vi "Update_Inlet_Temp_Profile.vi"(3 "Mode":T5, 5 "Traverse line In":T2 {"Carrier_2 Q (l/min)" format="%#.2f"; "Row Duration (mins)" format="%#.1f"; "Row No" min=0; "Trace Gas Concentration (%)" min=0.0 format="%#_4f"; "Carrier_1 Q (l/min)" format="%#.2f"; "Tunnel Speed" format="%#.2f"; "Start X" format="%#.2f"; "Start Y" format="%#.2f"; "Start Z" format="%#.2f"; "End X" format="%#.2f"; "End Y" format="%#.2f"; "End Z" format="%#.2f"; "Averaging time (min)" min=0.0 format="%#.2f"}) -> (0 "Error Message":string, 1 "Status":T1, 2 "Traverse line Out":T2 {"Carrier_2 Q (l/min)" format="%#.2f"; "Row Duration (mins)" format="%#.1f"; "Row No" min=0; "Trace Gas Concentration (%)" min=0.0 format="%#_4f"; "Carrier_1 Q (l/min)" format="%#.2f"; "Tunnel Speed" format="%#.2f"; "Start X" format="%#.2f"; "Start Y" format="%#.2f"; "Start Z" format="%#.2f"; "End X" format="%#.2f"; "End Y" format="%#.2f"; "End Z" format="%#.2f"; "Averaging time (min)" min=0.0 format="%#.2f"})   [LabVIEW 2015]
uses:
  Gen Trav/Traverse_cluster.ctl
  Gen Trav/Spacing.ctl
  Controls/Multi_run_mode.ctl
  Controls/User_Specific_mode.ctl
  Gen Trav/Multi_Run_Status.ctl
  <vilib>/Analysis/baseanly.llb/Mean (DBL).vi
  <vilib>/Analysis/NI_AALBase.lvlib
panel:
  out "Set Values":dbl[](array[numeric])
  out "Sub set":string[](array[string])=["EnFlo_Tunnel:Temp:Inlet_Y=0_Z=50", "EnFlo_Tunnel:Temp:Inlet_Y=0_Z=150", "EnFlo_Tunnel:Temp:Inlet_Y=0_Z=250", "EnFlo_Tunnel:Temp:Inlet_Y=0_Z=350", "EnFlo_Tunnel:Temp:Inlet_Y=0_Z=450", "EnFlo_Tunnel:Temp:Inlet_Y=0_Z=550", "EnFlo_Tunnel:Temp:Inlet_Y=0_Z=650", "EnFlo_Tunnel:Temp:Inlet_Y=0_Z=750", "EnFlo_Tunnel:Temp:Inlet_Y=0_Z=850", "EnFlo_Tunnel:Temp:Inlet_Y=0_Z=950", "EnFlo_Tunnel:Temp:Inlet_Y=0_Z=1050", "EnFlo_Tunnel:Temp:Inlet_Y=0_Z=1150", "EnFlo_Tunnel:Temp:Inlet_Y=0_Z=1250", "EnFlo_Tunnel:Temp:Inlet_Y=0_Z=1350", "EnFlo_Tunnel:Temp:Inlet_Y=0_Z=1450", "EnFlo_Tunnel:Chilled Water:Dem Temp"]
  out "Chilled water Dem Temp":dbl
  # "X           Y            Z"
  # "Start"
  # "End"
  # "X           Y            Z"
  # "Start"
  # "End"
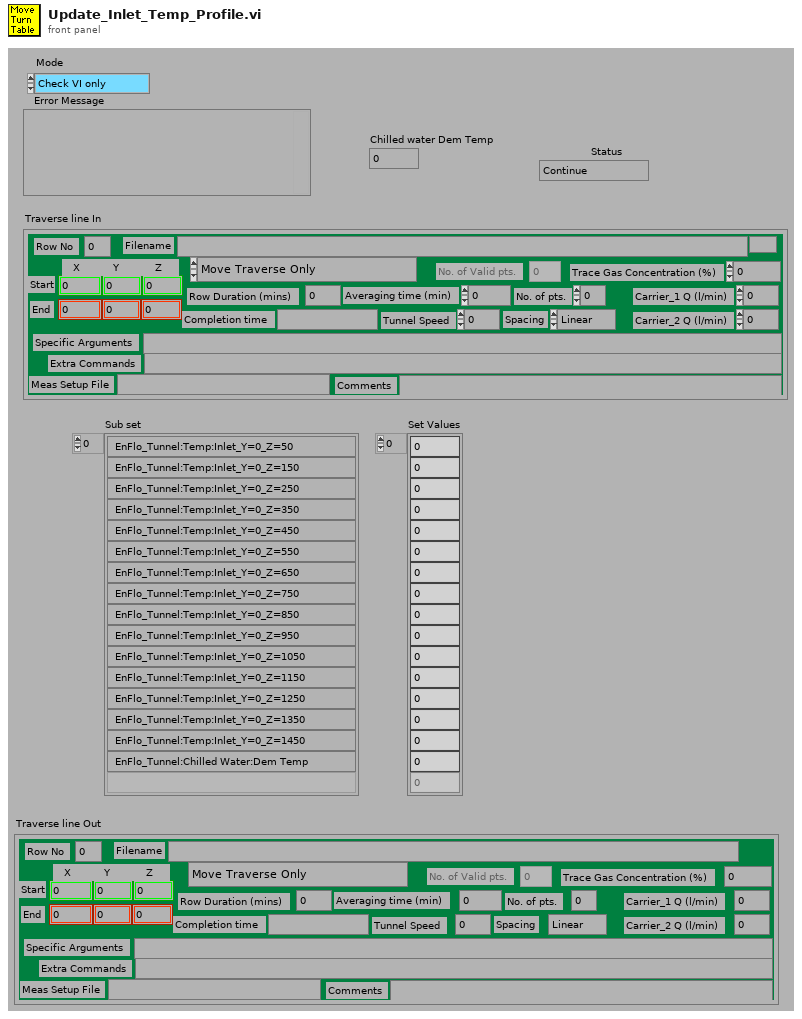
[diagram p1: front panel]
types:
  T1 = typedef "Multi_Run_Status.ctl" = enum16{"Continue", "Jump to Next Point", "Jump to Next Row", "Jump To Fall Back", "Terminate Run"}
  T2 = typedef "Traverse_cluster.ctl" = cluster{"Start X":sgl, "Start Y":sgl, "Start Z":sgl, "End X":sgl, "End Y":sgl, "End Z":sgl, "No. of pts.":i32, "Spacing":T3, "Filename":path, "Tunnel Speed":dbl, "Averaging time (min)":dbl, "Extra Commands":string, "Carrier_1 Q (l/min)":dbl, "Carrier_2 Q (l/min)":dbl, "Trace Gas Concentration (%)":dbl, "Specific Arguments":string, "Comments":string, "Row No":i32, "Row Type Selector":T4, "Completion time":string, "Row Duration (mins)":dbl, "No. of Valid pts.":i32, "Meas Setup File":string}
  T3 = typedef "Spacing.ctl" = enum16{"Linear", "Log", "Gauss", "Specified", "N/A"}
  T4 = typedef "Multi_run_mode.ctl" = enum16{"Move Traverse Only", "Set Tunnel Speed Only", "Set Source Only", "Set Measurement Conditions", "Single Measurement", "Vertical Profile", "Lateral Profile", "Longitudinal Profile", "Explore Volume", "Multi-Axis Profile", "Auto Calibrate", "Meas Fast FID Bkgnd", "Check Beam Power", "Scanning Valve Measurement", "Run VI Named:", "Set ADAM Ch", "Wait (minutes)", "Send Message", "Synchronize With:", "Fall Back to this Row", "Turn Off Row Repeating", "Blank Row", "Traverse 3D Volume"}
  T5 = typedef "User_Specific_mode.ctl" = enum16{"Check VI only", "Run VI"}
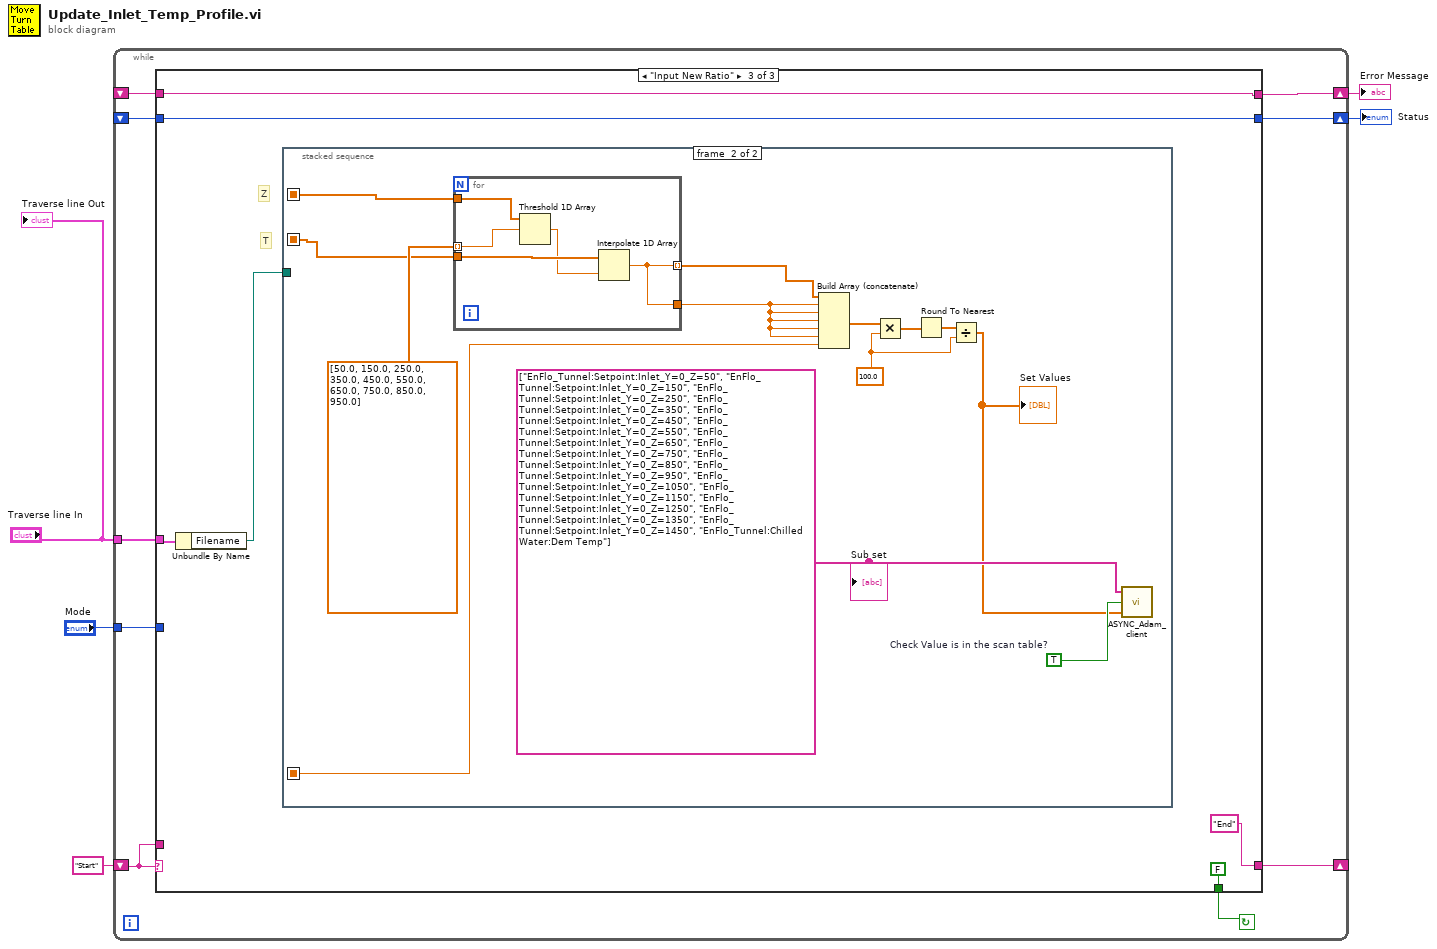
[diagram p0: block diagram]
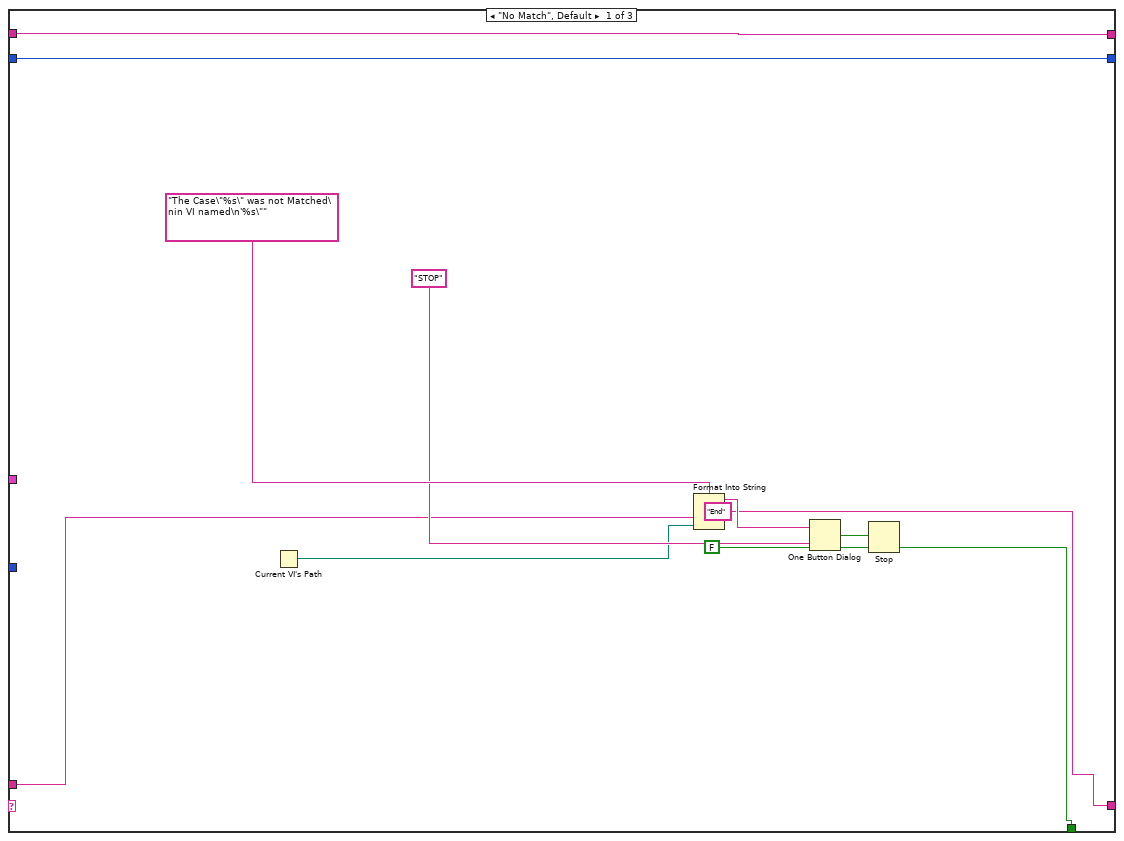
[diagram p2: hidden frame]
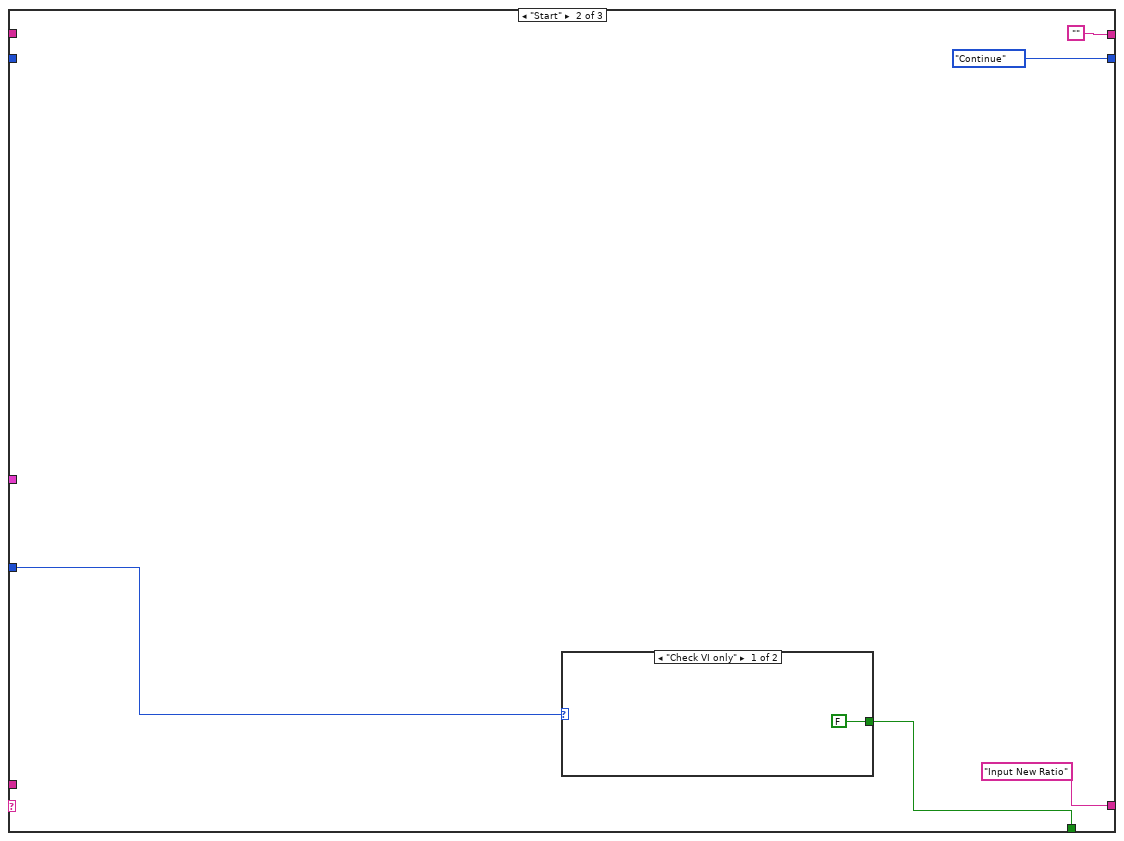
[diagram p3: hidden frame]
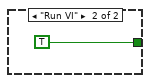
[diagram p4: hidden frame]
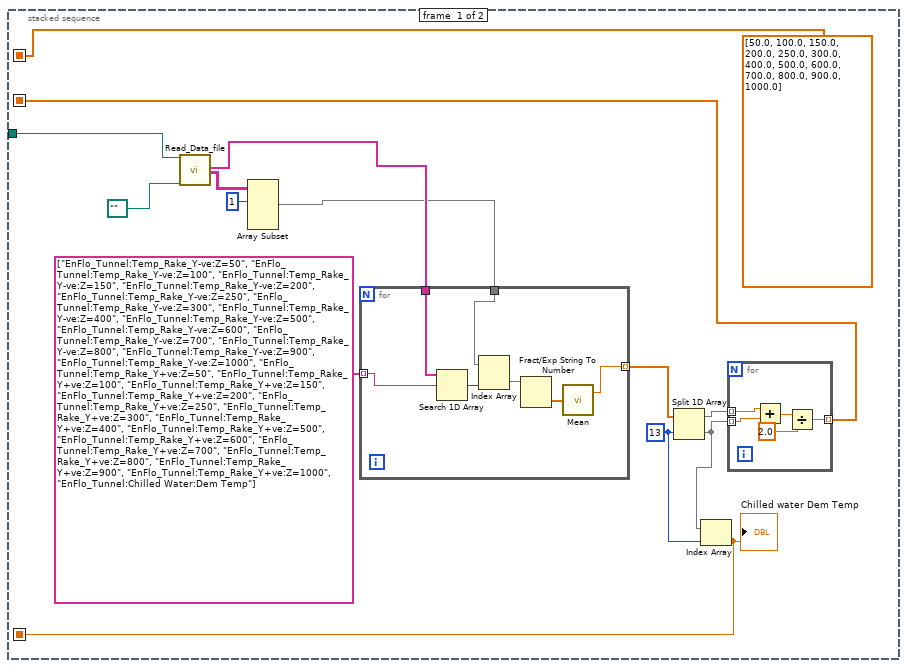
[diagram p5: hidden frame]
diagram:
  n1 = while {
    shift-left: _ -> [w7]
    shift-right: [w6] -> w2
    shift-left: _ -> [w10]
    shift-right: [w8] -> w3
    tunnel: "Traverse line In" -> [w13]
    tunnel: "Mode" -> [w14]
    shift-left: "Start" -> [w9]
    shift-right: [w11] -> _
    stop <- w12 continue-if-true
    n2 = case shown="\"Input New Ratio\"" w9 {
      tunnel: w13 -> [_ _ w35]
      tunnel: w14 -> [_ w28 _]
      tunnel: [FALSE ("Update Datum Powers?") w27 FALSE ("Update Datum Powers?")] -> w12
      tunnel: ["End" "Input New Ratio" "End"] -> w11
      tunnel: w10 -> [w19 _ w36]
      tunnel: [w19 "" w36] -> w8
      tunnel: w9 -> [w16 _ _]
      tunnel: w7 -> [w15 _ w37]
      tunnel: [w15 Multi_Run_Status."Continue" ("Status") w37] -> w6
      frame "No Match", Default {
        n3 = Current VI's Path() -> (path=w20:path)
        n4 = Format Into String(format string="The Case\"%s\" was not Matched\nin VI named\n'%s\"" ("Format String"), w16, w20) -> (resulting string=w23:string)  [unwired: 2 in, 1 out]
        n5 = One Button Dialog(message=w23, button name ("OK")="STOP") -> (true=w21:bool)
        n6 = Stop(stop? (T)=w21) -> ()
      }
      frame "Start" {
        n7 = case shown="\"Check VI only\"" w28 {
          tunnel: [FALSE ("Update Datum Powers?") TRUE ("Update Datum Powers?")] -> w27
          frame "Check VI only" {
          }
          frame "Run VI" {
          }
        }
      }
      frame "Input New Ratio" {
        # "T"
        # "Z"
        n8 = Unbundle By Name(w35) -> ("Filename"=w34:path)
        n9 = stacked-sequence {
          seq-local: [dbl[] [50.0, 100.0, 150.0, 200.0, 250.0, 300.0, 400.0, 500.0, 600.0, 700.0, 800.0, 900.0, 1000.0] ("second subarray") _] -> [_ w76]
          seq-local: [w42 _] -> [_ w74]
          seq-local: [w38 _] -> [_ w69]
          tunnel: w34 -> [w41 _]
          frame #0 {
            w39 = 13 ("index")
            n10 = call "Read_Data_file.vi"("Results file"=w41, "Template File"=path "") -> ("Ch names Out"=w50:string[], "Channel Values Out"=w48:string[][])  [unwired: 3 in, 13 out]
            n11 = Array Subset(array=w48, index (row)=1 ("index")) -> (w46:string[][])  [unwired: 3 in]
            n12 = for {
              tunnel: w50 -> [w63]
              tunnel: string[] ["EnFlo_Tunnel:Temp_Rake_Y-ve:Z=50", "EnFlo_Tunnel:Temp_Rake_Y-ve:Z=100", "EnFlo_Tunnel:Temp_Rake_Y-ve:Z=150", "EnFlo_Tunnel:Temp_Rake_Y-ve:Z=200", "EnFlo_Tunnel:Temp_Rake_Y-ve:Z=250", "EnFlo_Tunnel:Temp_Rake_Y-ve:Z=300", "EnFlo_Tunnel:Temp_Rake_Y-ve:Z=400", "EnFlo_Tunnel:Temp_Rake_Y-ve:Z=500", "EnFlo_Tunnel:Temp_Rake_Y-ve:Z=600", "EnFlo_Tunnel:Temp_Rake_Y-ve:Z=700", "EnFlo_Tunnel:Temp_Rake_Y-ve:Z=800", "EnFlo_Tunnel:Temp_Rake_Y-ve:Z=900", "EnFlo_Tunnel:Temp_Rake_Y-ve:Z=1000", "EnFlo_Tunnel:Temp_Rake_Y+ve:Z=50", "EnFlo_Tunnel:Temp_Rake_Y+ve:Z=100", "EnFlo_Tunnel:Temp_Rake_Y+ve:Z=150", "EnFlo_Tunnel:Temp_Rake_Y+ve:Z=200", "EnFlo_Tunnel:Temp_Rake_Y+ve:Z=250", "EnFlo_Tunnel:Temp_Rake_Y+ve:Z=300", "EnFlo_Tunnel:Temp_Rake_Y+ve:Z=400", "EnFlo_Tunnel:Temp_Rake_Y+ve:Z=500", "EnFlo_Tunnel:Temp_Rake_Y+ve:Z=600", "EnFlo_Tunnel:Temp_Rake_Y+ve:Z=700", "EnFlo_Tunnel:Temp_Rake_Y+ve:Z=800", "EnFlo_Tunnel:Temp_Rake_Y+ve:Z=900", "EnFlo_Tunnel:Temp_Rake_Y+ve:Z=1000", "EnFlo_Tunnel:Chilled Water:Dem Temp"] ("Sub set") -> [w62] mode=indexing
              tunnel: w46 -> [w61]
              tunnel: [w57] -> w45 mode=indexing
              n13 = Search 1D Array(1D array=w63, element=w62) -> (index of element=w60:i32)  [unwired: 1 in]
              n14 = Index Array(array=w61, index (col)=w60) -> (element=w59:string[])  [unwired: 1 in]
              n15 = Fract/Exp String To Number(string=w59) -> (number=w58:dbl[])  [unwired: 3 in, 1 out]
              n16 = call-poly <vilib>:"Mean.vi"("X"=w58) -> ("mean"=w57:dbl)  [unwired: 1 out]
            }
            n17 = Split 1D Array(array=w45, index=w39) -> (first subarray=w44:dbl[], second subarray=w40:dbl[])
            n18 = Index Array(array=w40, index=w39) -> (element=w38:dbl)
            "Chilled water Dem Temp" <- w38
            n19 = for {
              tunnel: w44 -> [w56] mode=indexing
              tunnel: w40 -> [w55] mode=indexing
              tunnel: [w52] -> w42 mode=indexing
              n20 = Add(x=w56, y=w55) -> (x+y=w54:dbl)
              n21 = Divide(x=w54, y=2.0) -> (x/y=w52:dbl)
            }
          }
          frame #1 {
            w65 = 100.0
            w70 = string[] ["EnFlo_Tunnel:Setpoint:Inlet_Y=0_Z=50", "EnFlo_Tunnel:Setpoint:Inlet_Y=0_Z=150", "EnFlo_Tunnel:Setpoint:Inlet_Y=0_Z=250", "EnFlo_Tunnel:Setpoint:Inlet_Y=0_Z=350", "EnFlo_Tunnel:Setpoint:Inlet_Y=0_Z=450", "EnFlo_Tunnel:Setpoint:Inlet_Y=0_Z=550", "EnFlo_Tunnel:Setpoint:Inlet_Y=0_Z=650", "EnFlo_Tunnel:Setpoint:Inlet_Y=0_Z=750", "EnFlo_Tunnel:Setpoint:Inlet_Y=0_Z=850", "EnFlo_Tunnel:Setpoint:Inlet_Y=0_Z=950", "EnFlo_Tunnel:Setpoint:Inlet_Y=0_Z=1050", "EnFlo_Tunnel:Setpoint:Inlet_Y=0_Z=1150", "EnFlo_Tunnel:Setpoint:Inlet_Y=0_Z=1250", "EnFlo_Tunnel:Setpoint:Inlet_Y=0_Z=1350", "EnFlo_Tunnel:Setpoint:Inlet_Y=0_Z=1450", "EnFlo_Tunnel:Chilled Water:Dem Temp"] ("Sub set")
            w71 = TRUE  # Check Value is in the scan table?
            n22 = for {
              tunnel: w76 -> [w81]
              tunnel: dbl[] [50.0, 150.0, 250.0, 350.0, 450.0, 550.0, 650.0, 750.0, 850.0, 950.0] ("second subarray") -> [w80] mode=indexing
              tunnel: w74 -> [w79]
              tunnel: [w77] -> w73 mode=indexing
              tunnel: [w77] -> w72
              n23 = Threshold 1D Array(2:w80, 3:w81) -> (0:w78:dbl)  [unwired: 1 in]
              n24 = Interpolate 1D Array(1:w78, 2:w79) -> (0:w77:dbl)
            }
            n25 = Build Array (concatenate)(w73, w72, w72, w72, w72, w72, w69) -> (w68:dbl[])
            n26 = Multiply(x=w68, y=w65) -> (x*y=w67:dbl[])
            n27 = Round To Nearest(number=w67) -> (nearest integer value=w66:dbl[])
            n28 = Divide(x=w66, y=w65) -> (x/y=w64:dbl[])
            "Set Values" <- w64
            n29 = call "ASYNC_Adam_client.vi"("Values"=w64, "Check Value is in the scan table?"=w71, "Channel Names"=w70) -> ()  [unwired: 2 out]
            "Sub set" <- w70
          }
        }
      }
    }
  }
  "Status" <- w2
  "Error Message" <- w3
  "Traverse line Out" <- "Traverse line In"
